vi "LabVIEW Pixel Font - VI Tree.vi"   [LabVIEW 2025]
uses:
  <vilib>/LabVIEW Icon API/Pixel Fonts/Picture Pixel Fonts.lvlib
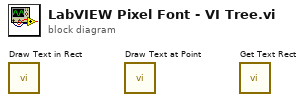
[diagram p0: block diagram]
diagram:
  n1 = call <vilib>:"Draw Text in Rect.vi"() -> ()  [unwired: 11 in, 1 out]
  n2 = call <vilib>:"Draw Text at Point.vi"() -> ()  [unwired: 10 in, 2 out]
  n3 = call <vilib>:"Get Text Rect.vi"() -> ()  [unwired: 9 in, 1 out]
